vi "Write_Analogue.vi"(2 "analogue value\nto write":u64, 3 "analogue channel\nto write":u8) -> (0 "Error Out":u8, 1 "Aborted":bool)   [LabVIEW 2017]
uses:
  <vilib>/rvi/Emulation/niFpgaEmulationIsFPGAContextNoSignature.vi
  <vilib>/rvi/DataTransferAndStorage/Container/Common/niFpgaContainerGetUniqueNameForEmu.vi
  <vilib>/rvi/Memory/Memory_Emulation/niFpgaMemoryEmulationCacheClearOnFirstRun.vi
  <vilib>/rvi/Memory/Memory_Emulation/nirvimemoryEmulationManagerCache_MakeExclusive.vi
  <vilib>/rvi/Memory/Memory_Emulation/niFpgaMemoryEmulationValidateCache.vi
  <vilib>/rvi/Memory/Memory_Emulation/nirvimemoryEmulationManagerCache_InsertValue.vi
  <vilib>/Utility/error.llb/Clear Errors.vi
  <vilib>/rvi/Memory/Memory_Emulation/nirvimemoryEmulationManagerCache_ReleaseExclusive.vi
  <vilib>/rvi/Memory/Memory_Emulation/nirvimemoryEmulationManagerCache_GetValue.vi
  <vilib>/rvi/Memory/Memory_Emulation/nirvimemoryEmulationManagerCache_SetValue.vi
  <vilib>/rvi/Emulation/niFpgaProcessEmulError.vi
  <vilib>/rvi/Emulation/niFpgaSctlEmulationGetInTimedLoop.vi
  <vilib>/rvi/eio/common/nirviEmuTemplateMethod_errors.vi
  <vilib>/rvi/DataTransferAndStorage/Container/XNode/niFpgaContainer.xnode
  <vilib>/rvi/DataTransferAndStorage/Register/Emulation/niFpgaRegisterEmulation.vi
  <vilib>/eio/EIONode/EIONode.xnode
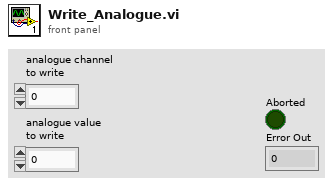
[diagram p1: front panel]
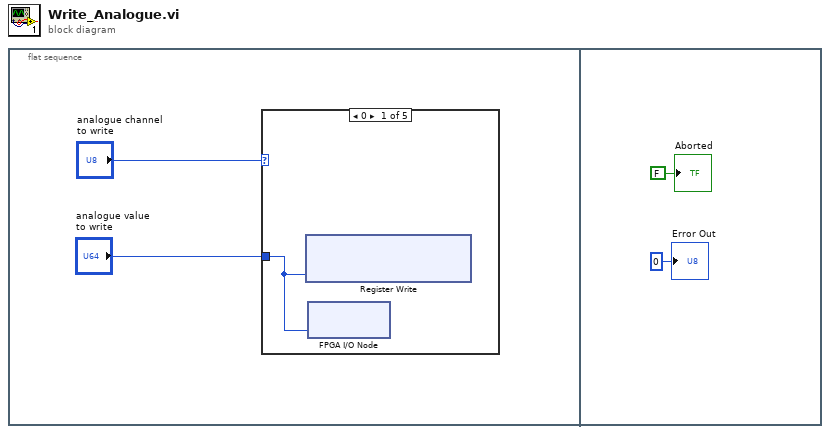
[diagram p0: block diagram]
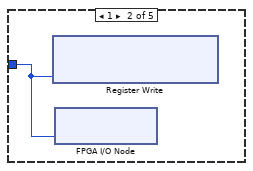
[diagram p2: hidden frame]
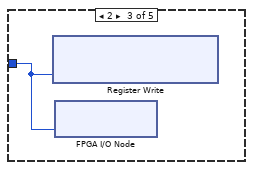
[diagram p3: hidden frame]
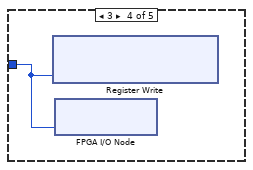
[diagram p4: hidden frame]
diagram:
  n1 = flat-sequence {
    frame #0 {
      n2 = case shown="0" "analogue channel\nto write" {
        tunnel: "analogue value\nto write" -> [w3 w4 w5 w6 _]
        frame 0 {
          n3 = xnode ("Register Write")("Data"=w3) -> ()  [unwired: 1 in, 1 out]
          n4 = xnode "FPGA I/O Node"("Z Stage"=w3) -> ()  [unwired: 1 in, 1 out]
        }
        frame 1 {
          n5 = xnode ("Register Write")("Data"=w4) -> ()  [unwired: 1 in, 1 out]
          n6 = xnode "FPGA I/O Node"("Mod1/AO1"=w4) -> ()  [unwired: 1 in, 1 out]
        }
        frame 2 {
          n7 = xnode ("Register Write")("Data"=w5) -> ()  [unwired: 1 in, 1 out]
          n8 = xnode "FPGA I/O Node"("Mod1/AO2"=w5) -> ()  [unwired: 1 in, 1 out]
        }
        frame 3 {
          n9 = xnode ("Register Write")("Data"=w6) -> ()  [unwired: 1 in, 1 out]
          n10 = xnode "FPGA I/O Node"("Mod1/AO3"=w6) -> ()  [unwired: 1 in, 1 out]
        }
        frame 4, Default {
        }
      }
    }
    frame #1 {
      "Aborted" <- FALSE
      "Error Out" <- u8 0
    }
  }
